vi "DiffDriveTrainSim_Update.vi"(6 "dT_Seconds":dbl=0.02, 11 "in DiffDriveTrainSim":T1 {"m_Motor"."Kt_NMPerAmp" format="%13.5p"; "m_Motor"."Kv_RadPerSecPerVolt" format="%13.5p"; "m_Motor"."R_Ohms" format="%13.5p"; "m_Motor"."FreeSpeed_RadPerSec" format="%13.5p"; "m_Motor"."FreeCurrent_Amps" format="%13.5p"; "m_Motor"."StallCurrent_Amps" format="%13.5p"; "m_Motor"."StallTorque_NM" format="%13.5p"; "m_Motor"."nominalVoltage_Volts" format="%13.5p"}) -> (0 "Error":bool, 3 "out DiffDriveTrainSim":T1 {"m_Motor"."Kt_NMPerAmp" format="%13.5p"; "m_Motor"."Kv_RadPerSecPerVolt" format="%13.5p"; "m_Motor"."R_Ohms" format="%13.5p"; "m_Motor"."FreeSpeed_RadPerSec" format="%13.5p"; "m_Motor"."FreeCurrent_Amps" format="%13.5p"; "m_Motor"."StallCurrent_Amps" format="%13.5p"; "m_Motor"."StallTorque_NM" format="%13.5p"; "m_Motor"."nominalVoltage_Volts" format="%13.5p"})   [LabVIEW 2019, in "Trajectory_Library.lvlib"]
doc: "Creates a new LINEAR SYSTEM data cluster with the specified values. \n\n\nInputs: \n - XXX -- XXX.\n\nOutputs:\n - XXX -- XXX."
uses:
  Trajectory_Library.lvlib
  DIFF_DRIVE_TRAIN_SIM.ctl
  LINEAR_SYSTEM.ctl
  <vilib>/Analysis/Matrix/Datatypes/RealMatrix.ctl
  DCMOTOR.CTL
  MatrixHelper_CoerceSize.vi
  MatBuilder_Create.vi
  DiffDriveTrainSim_GetDynamics.vi
  <vilib>/Analysis/1siggen.llb/Gaussian White Noise.vi
  <vilib>/Analysis/Matrix/Numeric/Add/Add - RM,RM.vi
  <vilib>/Analysis/Matrix/NI_Matrix.lvlib
panel:
  # "<States, 1>"
  # "<Outputs, 1>"
  # "<Inputs, 1>"
  # "<Outputs, 1>"
  # "<States,States>"
  # "<States,Inputs>"
  # "<Outputs,States>"
  # "<Outputs,Inputs>"
  # "<States, 1>"
  # "<Outputs, 1>"
  # "<Inputs, 1>"
  # "<Outputs, 1>"
  # "<States,States>"
  # "<States,Inputs>"
  # "<Outputs,States>"
  # "<Outputs,Inputs>"
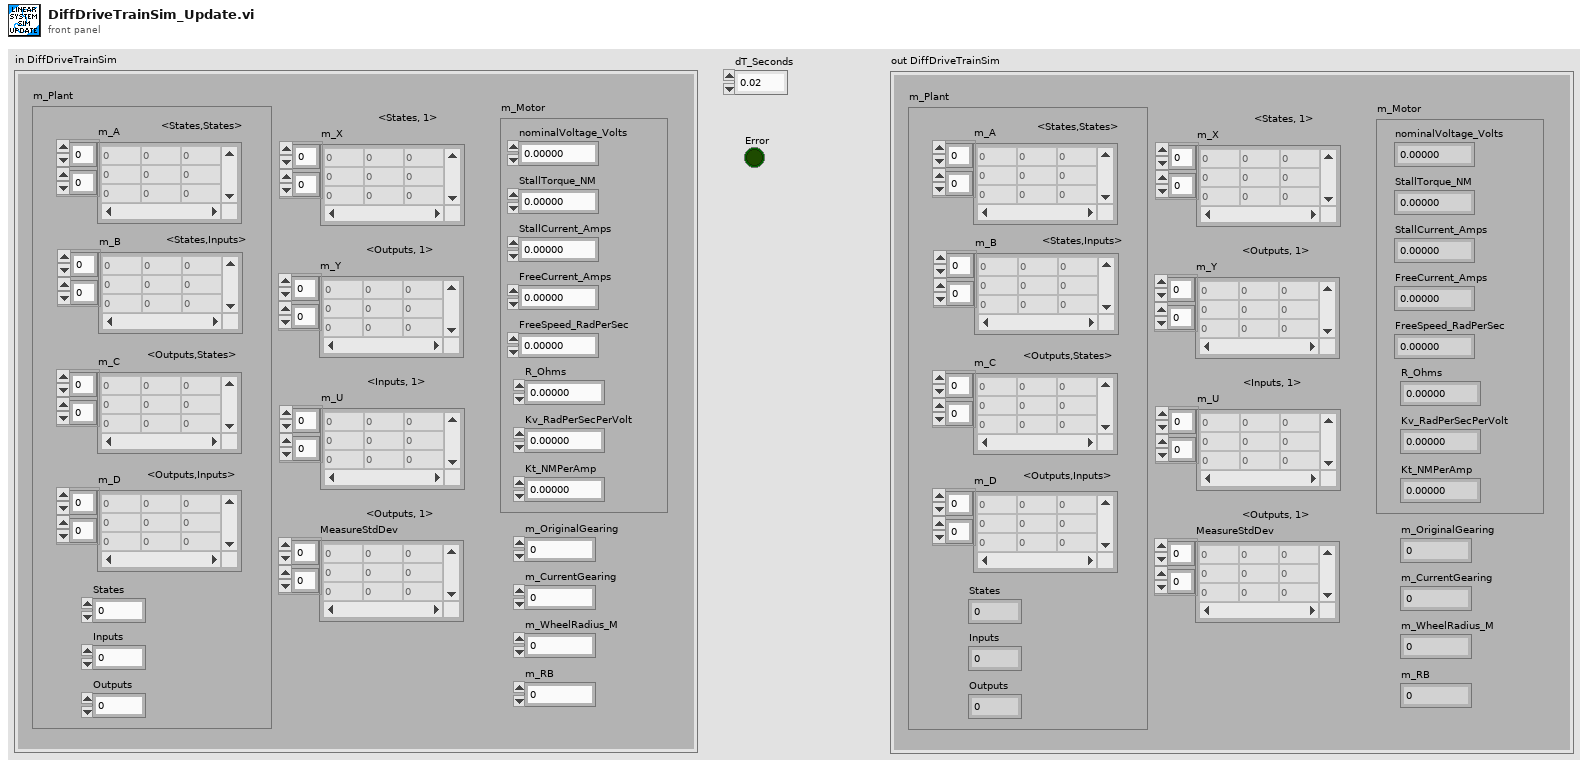
[diagram p1: front panel]
types:
  T1 = typedef "Trajectory_Library.lvlib/DIFF_DRIVE_TRAIN_SIM.ctl" = cluster{"m_Plant":T2, "m_X":T3, "m_Y":T3, "m_U":T3, "MeasureStdDev":T3, "m_Motor":T4, "m_OriginalGearing":dbl, "m_CurrentGearing":dbl, "m_WheelRadius_M":dbl, "m_RB":dbl}
  T2 = typedef "Trajectory_Library.lvlib/LINEAR_SYSTEM.ctl" = cluster{"m_A":T3, "m_B":T3, "m_C":T3, "m_D":T3, "States":i32, "Inputs":i32, "Outputs":i32}
  T3 = typedef "NI_Matrix.lvlib/RealMatrix.ctl" = dbl[][]
  T4 = typedef "Trajectory_Library.lvlib/DCMOTOR.CTL" = cluster{"nominalVoltage_Volts":dbl, "StallTorque_NM":dbl, "StallCurrent_Amps":dbl, "FreeCurrent_Amps":dbl, "FreeSpeed_RadPerSec":dbl, "R_Ohms":dbl, "Kv_RadPerSecPerVolt":dbl, "Kt_NMPerAmp":dbl}
  T5 = cluster{"m_A":T3, "m_B":T3, "m_CurrentGearing":dbl, "m_OriginalGearing":dbl, "m_RB":dbl}
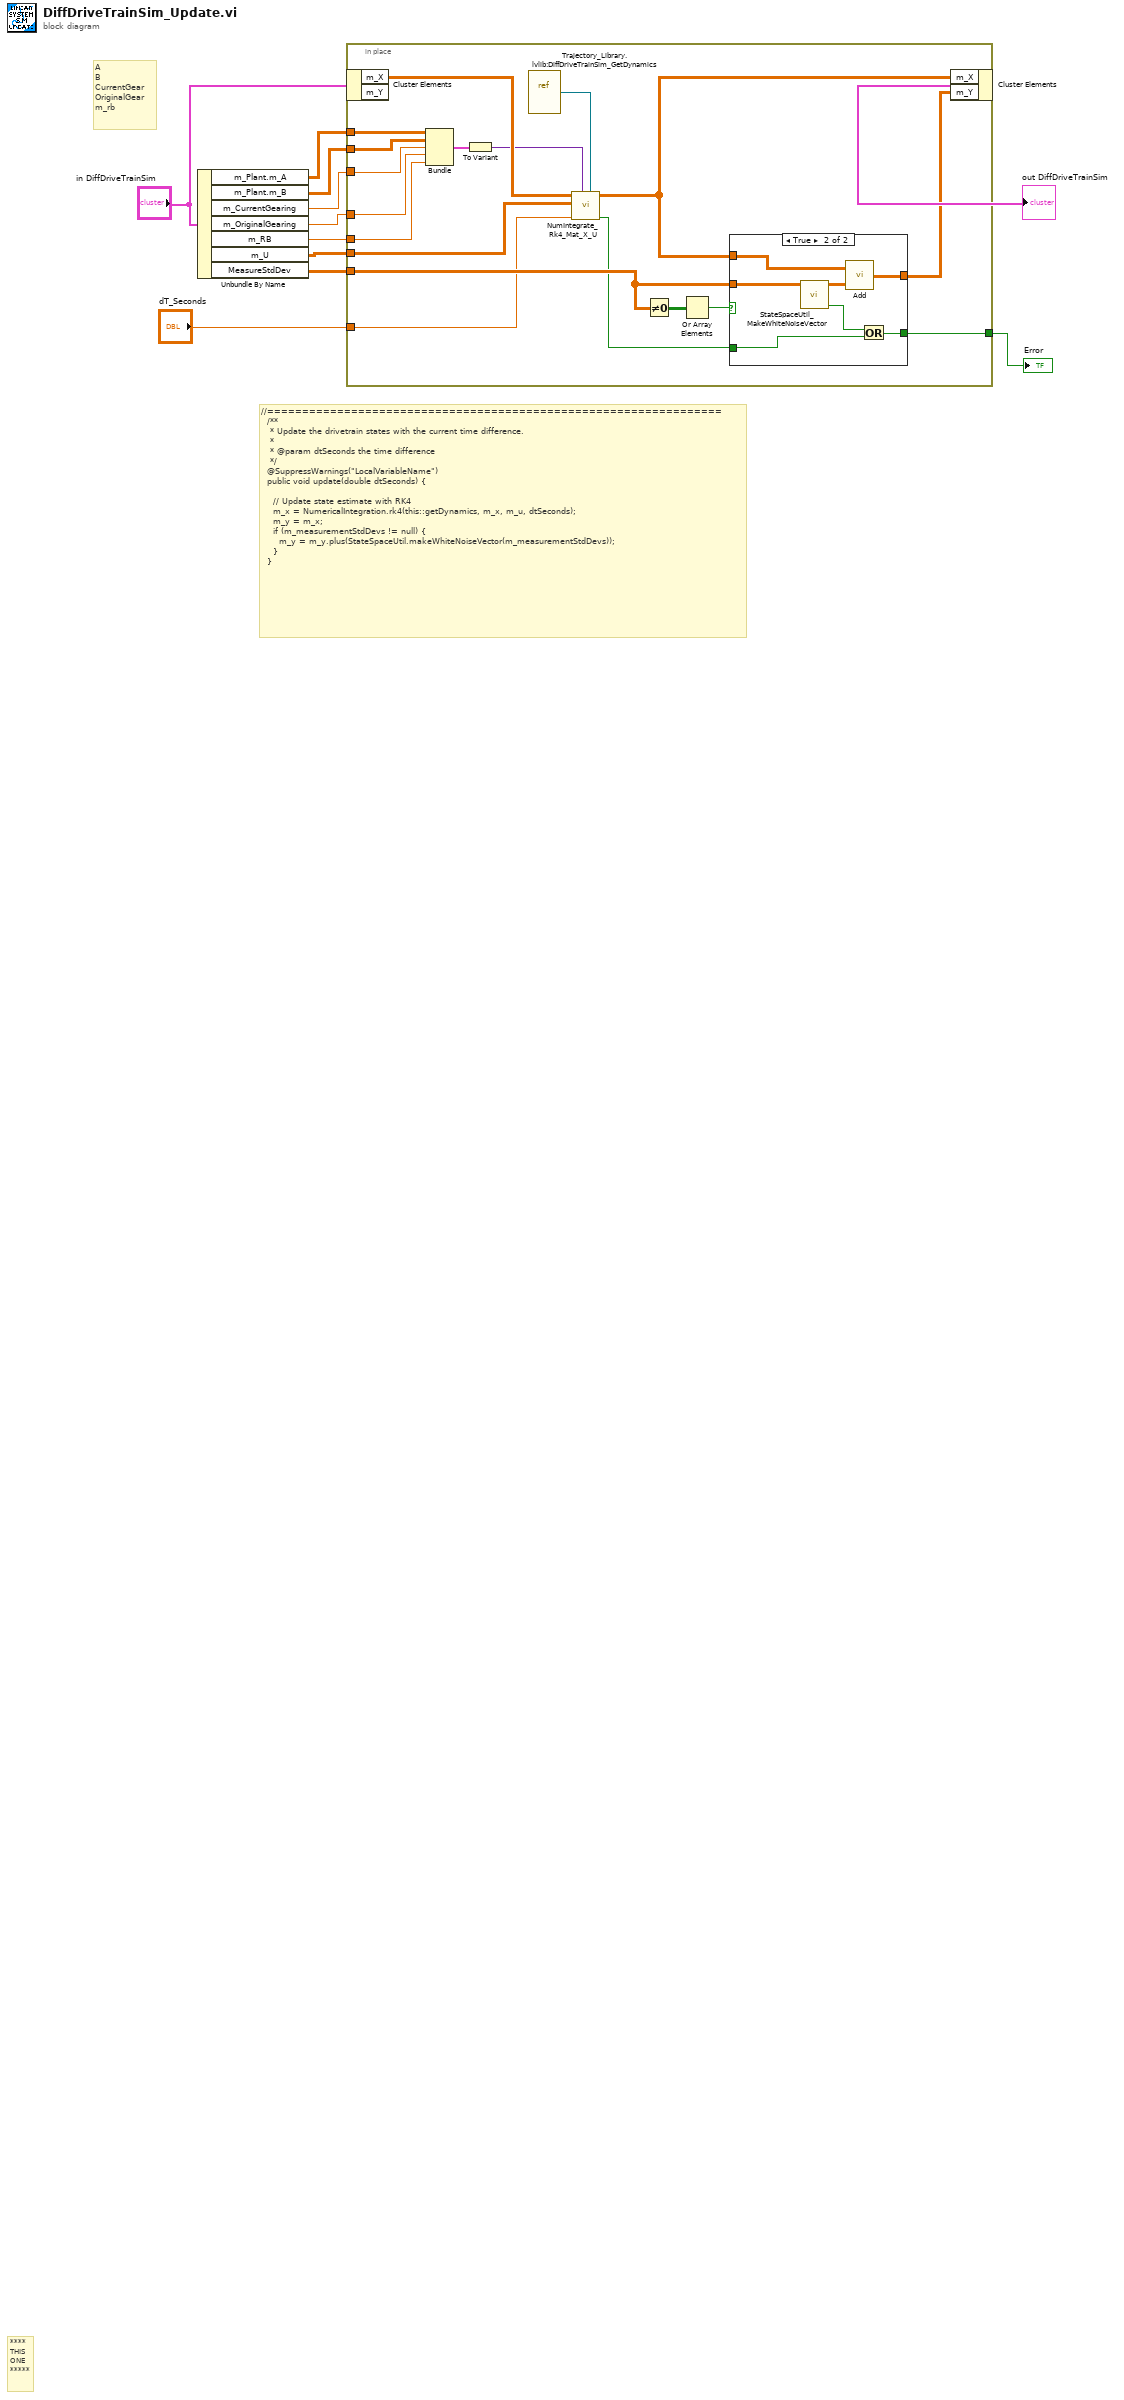
[diagram p0: block diagram]
diagram:
  # "A\nB\nCurrentGear\nOriginalGear\nm_rb"
  # "//=================================================================\n  /**\n   * Update the drivetrain states with the current time difference.\n   *\n   * @param dtSeconds the time difference\n   */\n  @SuppressWarnings(\"LocalVariableName\")\n  public void update(double dtSeconds) {\n\n    // Update state estimate with RK4\n    m_x = NumericalIntegration.rk4(this::getDynamics, m_x, m_u, dtSeconds);\n    m_y = m_x;\n    if (m_measurementStdDevs != null) {\n      m_y = m_y.plus(StateSpaceUtil.makeWhiteNoiseVector(m_measurementStdDevs));\n    }\n  }"
  # "****\nTHIS\nONE\n*****"
  n1 = Unbundle By Name("in DiffDriveTrainSim") -> ("m_Plant.m_A"=w6:T3, "m_Plant.m_B"=w5:T3, "m_CurrentGearing"=w4:dbl, "m_OriginalGearing"=w3:dbl, "m_RB"=w2:dbl, "m_U"=w11:T3, "MeasureStdDev"=w7:T3)
  n2 = in-place {
    in-place-border: w11 -> [w24]
    in-place-border: "dT_Seconds" -> [w25]
    in-place-border: w7 -> [w29]
    in-place-border: w6 -> [w19]
    in-place-border: w5 -> [w18]
    in-place-border: w4 -> [w17]
    in-place-border: w3 -> [w16]
    in-place-border: w2 -> [w15]
    in-place-border: [w12] -> w1
    n3 = in-place-cluster #1("in DiffDriveTrainSim") -> ("m_X"=w22:T3)  [unwired: 1 out]
    n4 = Bundle("m_A"=w19, "m_B"=w18, "m_CurrentGearing"=w17, "m_OriginalGearing"=w16, "m_RB"=w15) -> (w14:T5)  [unwired: 1 in]
    n5 = To Variant(anything=w14) -> (Variant=w20:variant)
    n6 = vi-ref "Trajectory_Library.lvlib:DiffDriveTrainSim_GetDynamics.vi"() -> (w21:refnum<vi>)
    n7 = call "NumIntegrate_Rk4_Mat_X_U.vi"("NumInt_RK4_Func_Type"=w21, "PassedData"=w20, "dT_Seconds"=w25, "U"=w24, "X"=w22) -> ("Error"=w13:bool, "OUTPUT"=w23:T3)  [unwired: 5 in]
    n8 = Not Equal To 0?(x=w29) -> (x != 0?=w28:bool[][])
    n9 = Or Array Elements(Boolean array=w28) -> (logical OR=w27:bool)
    n10 = case shown="True" w27 {
      tunnel: w29 -> [_ w38]
      tunnel: w23 -> [w31 w36]
      tunnel: [w31 w35] -> w26
      tunnel: w13 -> [w30 w33]
      tunnel: [w30 w32] -> w12
      frame False {
      }
      frame True {
        n11 = call "StateSpaceUtil_MakeWhiteNoiseVector.vi"("StdDevs"=w38) -> ("Size Coerced"=w34:bool, "WhiteNoise"=w37:T3)  [unwired: 9 in]
        n12 = call-poly <vilib>:"Add.vi"("Real Matrix B"=w37, "Real Matrix A"=w36) -> ("A + B"=w35:T3)
        n13 = Or(x=w34, y=w33) -> (x .or. y?=w32:bool)
      }
    }
    n14 = in-place-cluster #1("m_X"=w23, "m_Y"=w26) -> (→"out DiffDriveTrainSim":T1)
  }
  "Error" <- w1
